vi "DSC_ArchiveTrace.vi"   [LabVIEW 2013]
uses:
  <vilib>/lvdsc/NI_DSC.lvlib
types:
  T1 = cluster{"show status bar (T)":bool, "compact (T)":bool, "use * as wildcard (F)":bool, "delete data from source database (F)":bool}
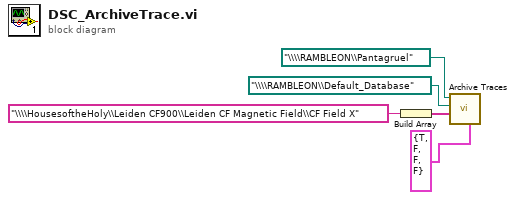
[diagram p0: block diagram]
diagram:
  n1 = Build Array("\\\\HousesoftheHoly\\Leiden CF900\\Leiden CF Magnetic Field\\CF Field X") -> (w1:string[])
  n2 = call <vilib>:"Archive Traces.vi"("options"=T1 {"show status bar (T)"=TRUE, "compact (T)"=FALSE, "use * as wildcard (F)"=FALSE, "delete data from source database (F)"=FALSE}, "trace names"=w1, "destination database URL"=path "\\\\RAMBLEON\\Default_Database", "source database URL"=path "\\\\RAMBLEON\\Pantagruel") -> ()  [unwired: 5 in, 3 out]
